vi "FlattenToString.vi"(8 "error in (no error)":errorcluster, 11 "dvotAFTKinetics in":refnum<class "dvotAFTKinetics.lvclass">) -> (0 "error out":errorcluster, 2 "String out":string, 3 "dvotAFTKinetics out":refnum<class "dvotAFTKinetics.lvclass">)   [LabVIEW 2012, in "dvotAFTKinetics.lvclass"]
uses:
  dvotAFTKinetics.lvclass
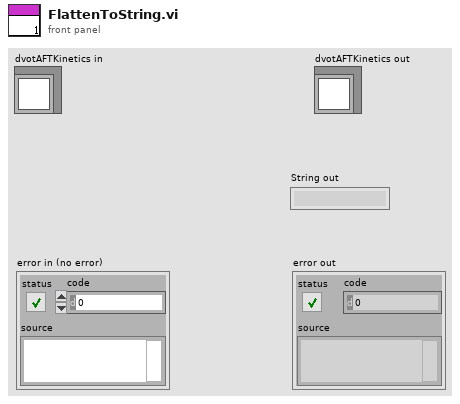
[diagram p1: front panel]
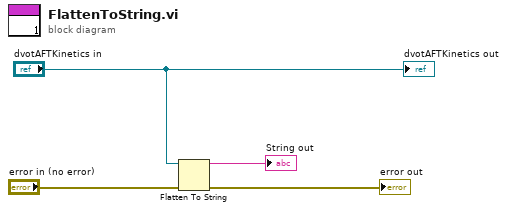
[diagram p0: block diagram]
diagram:
  n1 = Flatten To String(anything="dvotAFTKinetics in", error in (no error)="error in (no error)") -> (data string=→"String out":string, error out=→"error out":errorcluster)  [unwired: 2 in, 1 out]
  "dvotAFTKinetics out" <- "dvotAFTKinetics in"
